vi "BotSpeak_COMWrite.vi"(2 "COM Port":u8(slide)=2 scale=1.0..3.0, 3 "string":string, 4 "Bot Settings":T1) -> (0 "response":string, 1 "Bot Settings 2":T1)   [LabVIEW 2014]
doc: "Writes the specified \"string\" to the specified \"COM Port\"."
uses:
  <userlib>/botspeakLib/VIs/Direct/BotSpeak_Control.ctl
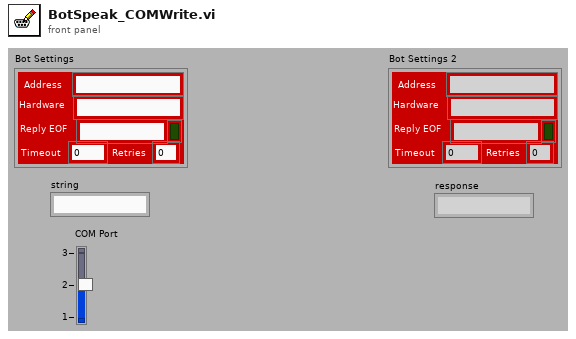
[diagram p1: front panel]
types:
  T1 = typedef "BotSpeak_Control.ctl" = cluster{"Address":string, "Reply EOF":string, "Hardware":string, "Retries":i8, "Timeout":i32, "Open?":bool}
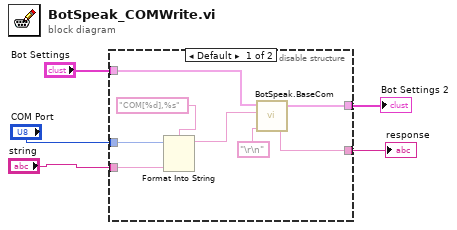
[diagram p0: block diagram]
diagram:
  n1 = disable-structure shown="Default" {
    disable-tunnel: "COM Port" -> [w13 _]
    disable-tunnel: "string" -> [w12 _]
    disable-tunnel: "Bot Settings" -> [w10 _]
    disable-tunnel: [w9 _] -> w2
    disable-tunnel: [w7 _] -> w1
    frame condition #0 {
      n2 = Format Into String(format string="COM[%d],%s" ("command"), w13, w12) -> (resulting string=w8:string)  [unwired: 2 in, 1 out]
      n3 = call <userlib>:"BotSpeak.BaseCom.vi"("Termination"="\r\n", "command"=w8, "Bot Settings in"=w10) -> ("response"=w7:string, "Bot Settings out"=w9:T1)  [unwired: 2 in]
    }
    frame condition #1 (active) {
    }
  }
  "response" <- w1
  "Bot Settings 2" <- w2
